vi "Init.vi"() -> (3 "Teardown Error Msg out":refnum<class "Teardown Error Msg.lvclass">)   [LabVIEW 2020, in "jettl.lvlib" / "Teardown Error Msg.lvlib" / "Teardown Error Msg.lvclass"]
uses:
  Teardown Error Msg.lvclass
  Sender/Sender/Sender.lvclass
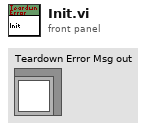
[diagram p1: front panel]
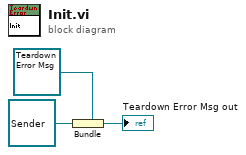
[diagram p0: block diagram]
diagram:
  n1 = Bundle "Bundle"(cluster=refnum<class "Teardown Error Msg.lvclass"> refnum ("Destroy Msg in"), refnum<class "Sender.lvclass"> refnum ("Sender")) -> (→"Teardown Error Msg out":refnum<class "Teardown Error Msg.lvclass">)
